vi "DB Select.vi"(4 "Group By":string, 6 "Orderby":string, 7 "table Name":string, 8 "error in (no error)":errorcluster, 9 "Column Name":string[](array[string]), 10 "Where Condition":string, 11 "Db Reference":refnum<k24>) -> (0 "error out":errorcluster, 2 "Data":string[][](array[string]), 3 "Db Reference":refnum<k24>)   [LabVIEW 2020]
uses:
  D:/Labview/Auto Run Screen/Source Code/Database/Support/dbquery.dll
  Support/dbquery.dll
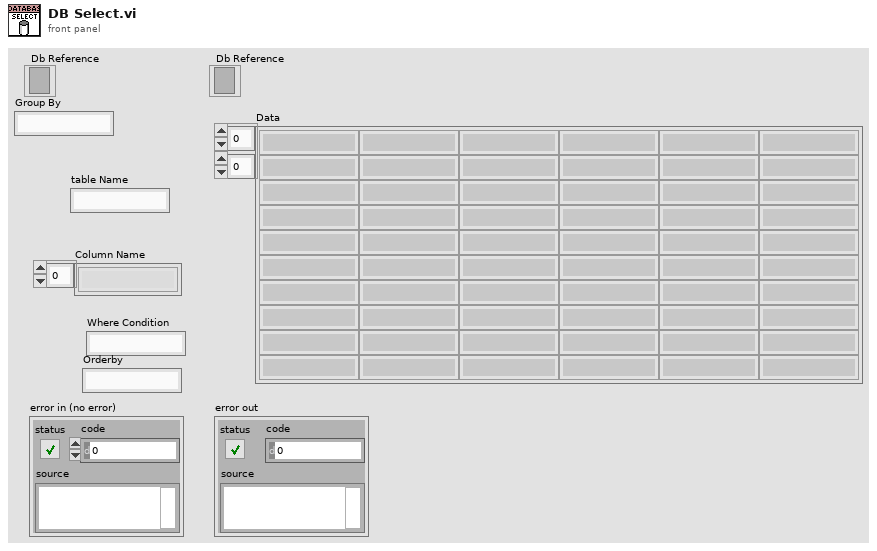
[diagram p1: front panel]
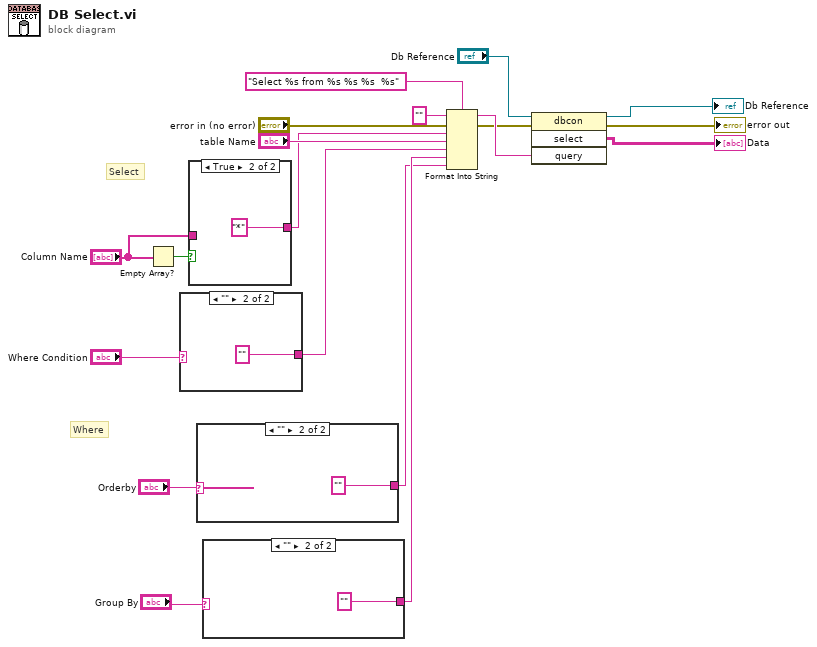
[diagram p0: block diagram]
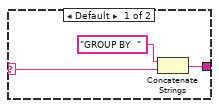
[diagram p2: hidden frame]
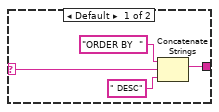
[diagram p3: hidden frame]
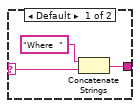
[diagram p4: hidden frame]
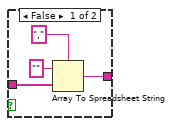
[diagram p5: hidden frame]
diagram:
  # "Where"
  # "Select"
  n1 = Empty Array?(array="Column Name") -> (empty?=w15:bool)
  n2 = case shown="\"\"" "Where Condition" {
    selector: "Where Condition" -> [w20 _]
    tunnel: [w21 ""] -> w8
    frame Default {
      n3 = Concatenate Strings("Where  ", w20) -> (w21:string)
    }
    frame "" {
    }
  }
  n4 = case shown="True" w15 {
    tunnel: [w24 "*"] -> w14
    tunnel: "Column Name" -> [w27 _]
    frame False {
      n5 = Array To Spreadsheet String(delimiter (Tab)=",", array=w27, 3:"" ("format string")) -> (spreadsheet string=w24:string)
    }
    frame True {
    }
  }
  n6 = case shown="\"\"" "Orderby" {
    selector: "Orderby" -> [w30 _]
    tunnel: [w31 ""] -> w1
    frame Default {
      n7 = Concatenate Strings("ORDER BY  ", w30, " DESC") -> (w31:string)
    }
    frame "" {
    }
  }
  n8 = case shown="\"\"" "Group By" {
    selector: "Group By" -> [w34 _]
    tunnel: [w35 ""] -> w2
    frame Default {
      n9 = Concatenate Strings("GROUP BY  ", w34) -> (w35:string)
    }
    frame "" {
    }
  }
  n10 = Format Into String(format string="Select %s from %s %s %s  %s", initial string="", error in="error in (no error)", w14, "table Name", w8, w2, w1) -> (resulting string=w12:string, error out=w10:errorcluster)
  n11 = invoke class="dbcon" method="select"(reference="Db Reference", error in=w10, "query"=w12) -> (reference out=→"Db Reference":refnum<k24>, error out=→"error out":errorcluster, "select"=→"Data":string[][])  [unwired: 1 in, 1 out]
